vi "create_object.vi"(1 "Run Data":T1) -> (0 "Run":refnum<class "Run.lvclass">)   [LabVIEW 2020, in "Run.lvclass"]
uses:
  Run.lvclass
  Run Data.ctl
  Run.lvclass/Run.ctl
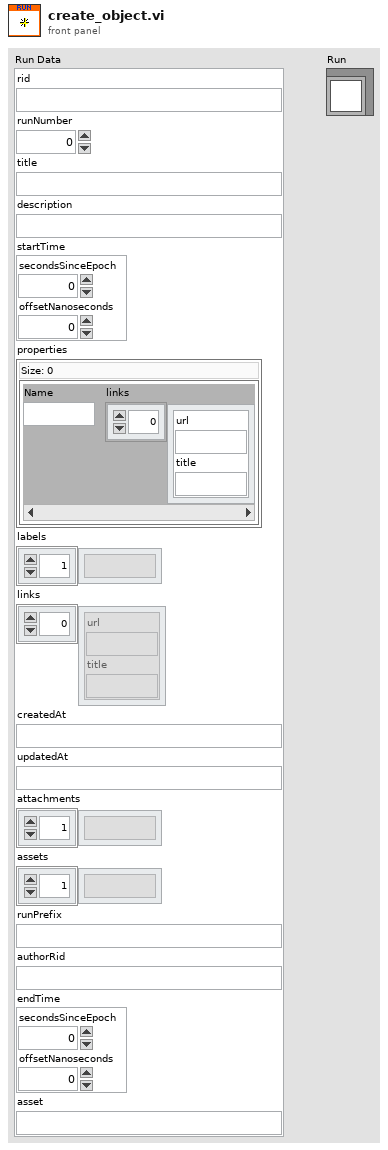
[diagram p1: front panel]
types:
  T1 = typedef "Run.lvclass/Run Data.ctl" = cluster{"rid":string, "runNumber":i32, "title":string, "description":string, "startTime":cluster{"secondsSinceEpoch":i32, "offsetNanoseconds":i32}, "properties":map{string, cluster{"url":string, "title":string}[]}, "labels":string[], "links":cluster{"url":string, "title":string}[], "createdAt":string, "updatedAt":string, "attachments":string[], "assets":string[], "runPrefix":string, "authorRid":string, "endTime":cluster{"secondsSinceEpoch":i32, "offsetNanoseconds":i32}, "asset":string}
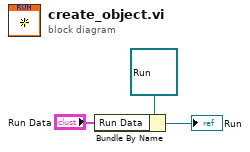
[diagram p0: block diagram]
diagram:
  n1 = Bundle By Name(cluster=refnum<class "Run.lvclass"> refnum ("Run"), "Run Data"="Run Data") -> (→"Run":refnum<class "Run.lvclass">)
